vi "Standard Teleop Emulator.vi"(11 "device ID":refnum<k1>) -> (3 "Robot Velocities":T1)   [LabVIEW 2025]
uses:
  swerve-template/Type Definitions/Data/Robot Velocities.ctl
panel:
  in  "Max Velocities":cluster{"vx":dbl, "vy":dbl, "w":dbl}={"vx"=10.0, "vy"=10.0, "w"=180.0}
  in  "Deadband":dbl=0.1
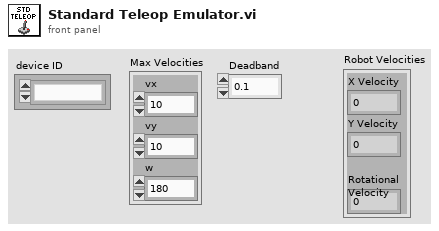
[diagram p1: front panel]
types:
  T1 = typedef "Robot Velocities.ctl" = cluster{"X Velocity":dbl, "Y Velocity":dbl, "Rotational \nVelocity":dbl}
  T2 = cluster{"X axis":i32, "Y axis":i32, "Z axis":i32, "X axis rotation":i32, "Y axis rotation":i32, "Z axis rotation":i32, "U axis":i32, "V axis":i32}
  T3 = cluster{"X axis":dbl, "Y axis":dbl, "Z axis":dbl, "X axis rotation":dbl, "Y axis rotation":dbl, "Z axis rotation":dbl, "U axis":dbl, "V axis":dbl}
  T4 = cluster{"X axis":dbl, dbl, "X axis rotation":dbl}
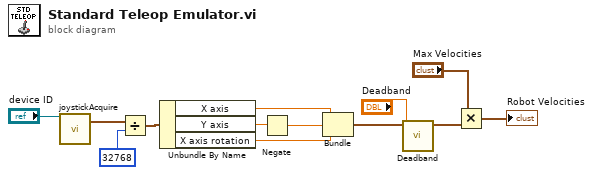
[diagram p0: block diagram]
diagram:
  n1 = call <vilib>:"joystickAcquire.vi"("device ID"="device ID") -> ("axis info"=w9:T2)  [unwired: 14 in, 4 out]
  n2 = Divide(x=w9, y=32768 ("X axis")) -> (x/y=w7:T3)
  n3 = Unbundle By Name(w7) -> ("X axis"=w5:dbl, "Y axis"=w2:dbl, "X axis rotation"=w4:dbl)
  n4 = Negate(x=w2) -> (-x=w1:dbl)
  n5 = Bundle("X axis"=w5, w1, "X axis rotation"=w4) -> (w13:T4)  [unwired: 1 in]
  n6 = call "Deadband.vi"("Deadband Info"="Deadband", "Robot Velocities"=w13) -> ("Adjusted Robot Velocities"=w11:T1)  [unwired: 8 in, 1 out]
  n7 = Multiply(x="Max Velocities", y=w11) -> (x*y=→"Robot Velocities":T1)
